vi "Set Speed.vi"(8 "error in (no error)":errorcluster, 10 "speed":dbl, 11 "VICI Settings":T1) -> (0 "error out":errorcluster, 1 "Connection Error":bool, 3 "VICI Settings":T1)   [LabVIEW 2018, in "VICI M50 Party Mode.lvlib"]
uses:
  VICI M50 Party Mode.lvlib
  Settings Cluster.ctl
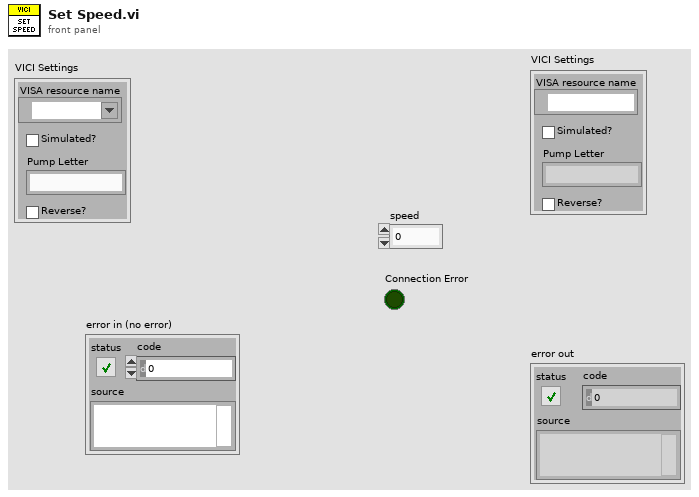
[diagram p1: front panel]
types:
  T1 = typedef "VICI M50 Party Mode.lvlib/Settings Cluster.ctl" = cluster{"VISA resource name":refnum<visa-resource-name>, "Simulated?":bool, "Pump Letter":string, "Reverse?":bool}
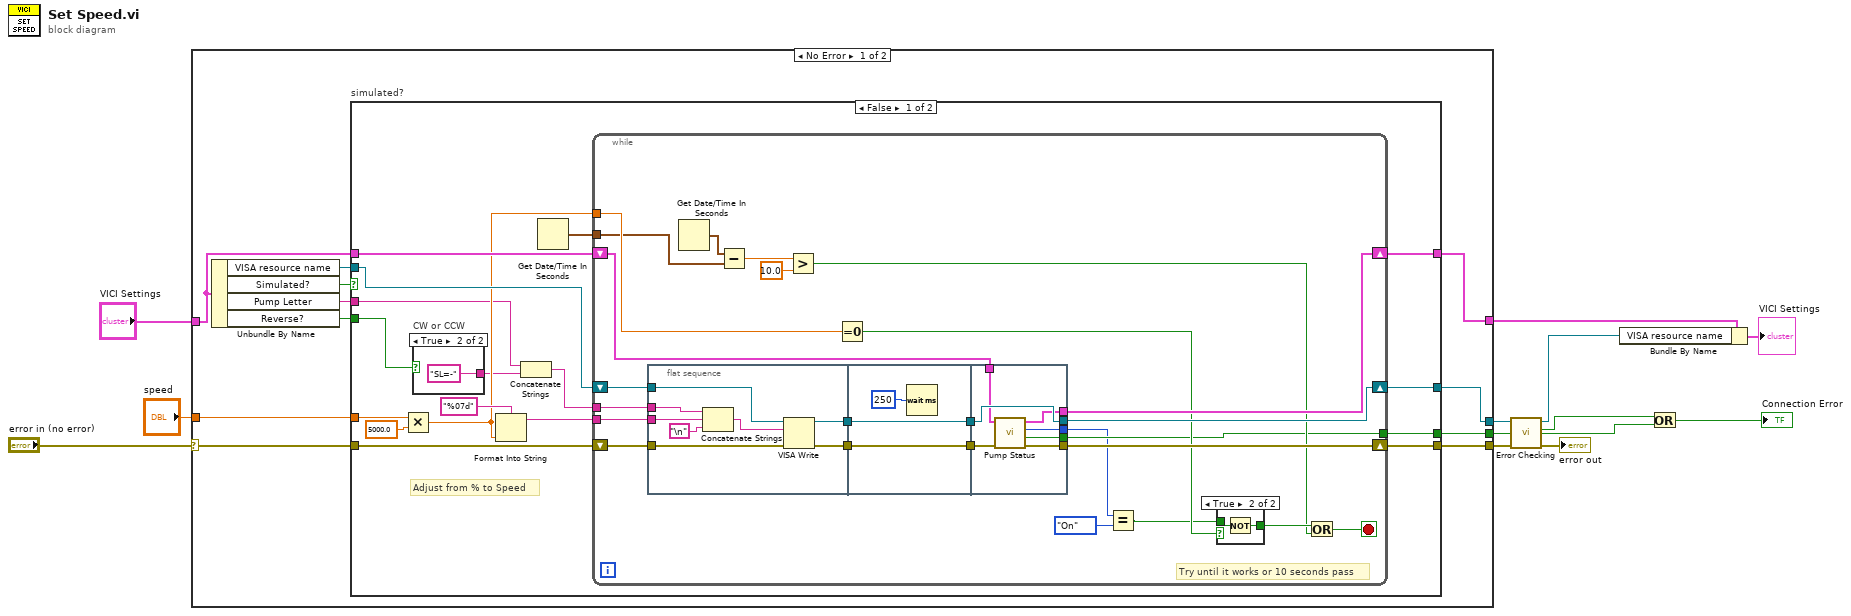
[diagram p0: block diagram]
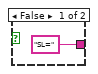
[diagram p3: hidden frame]
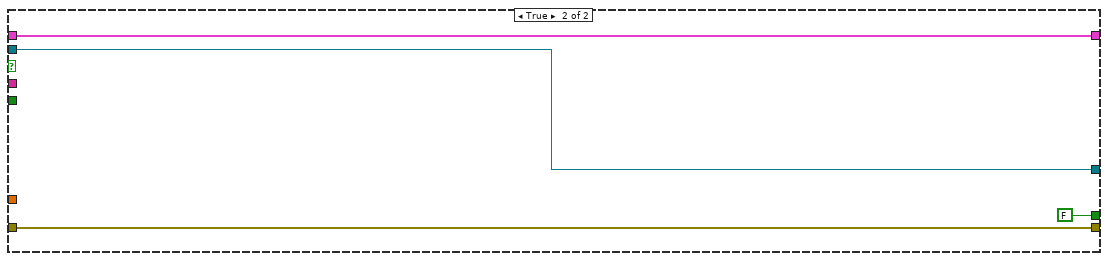
[diagram p4: hidden frame]
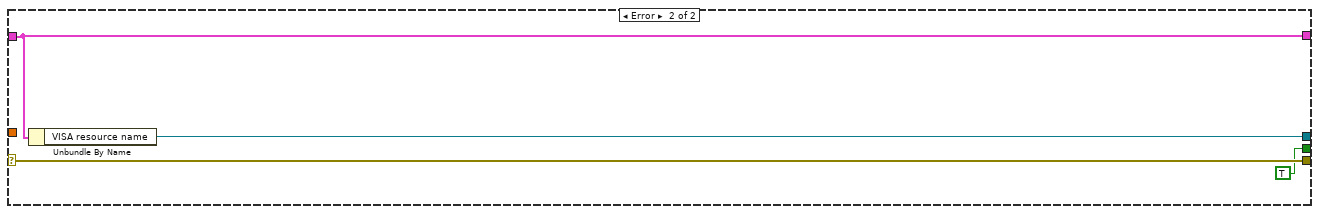
[diagram p5: hidden frame]
diagram:
  n1 = case shown="No Error" "error in (no error)" {
    selector: "error in (no error)" -> [w20 w96]
    tunnel: [w15 w95] -> w5
    tunnel: "VICI Settings" -> [w16 w95]
    tunnel: "speed" -> [w19 _]
    tunnel: [w18 w94] -> w9
    tunnel: [w17 w96] -> w8
    tunnel: [w14 TRUE ("Connection Error")] -> w3
    frame No Error {
      n2 = Unbundle By Name(w16) -> ("VISA resource name"=w22:refnum<visa-resource-name>, "Simulated?"=w21:bool, "Pump Letter"=w13:string, "Reverse?"=w23:bool)
      n3 = case "simulated?" shown="False" w21 {
        tunnel: [w38 w92] -> w18
        tunnel: w22 -> [w40 w92]
        tunnel: w20 -> [w39 w91]
        tunnel: [w37 w91] -> w17
        tunnel: w23 -> [w36 _]
        tunnel: w19 -> [w34 _]
        tunnel: w16 -> [w31 w90]
        tunnel: [w30 w90] -> w15
        tunnel: [w27 FALSE ("Connection Error")] -> w14
        tunnel: w13 -> [w24 _]
        frame False {
          # "Adjust from % to Speed"
          n4 = Multiply(x=w34, y=5000.0) -> (x*y=w29:dbl)
          n5 = case "CW or CCW" shown="True" w36 {
            tunnel: ["SL=" ("string") "SL=-" ("string")] -> w26
            frame False {
            }
            frame True {
            }
          }
          n6 = Format Into String(format string="%07d", w29) -> (resulting string=w33:string)  [unwired: 2 in, 1 out]
          n7 = Concatenate Strings(w24, w26) -> (w25:string)
          n8 = Get Date/Time In Seconds() -> (seconds since 1Jan1904=w28:timestamp)
          n9 = while {
            tunnel: w25 -> [w58]
            tunnel: w33 -> [w57]
            shift-right: [w60] -> w38
            shift-left: w40 -> [w45]
            shift-right: [w59] -> w37
            shift-left: w39 -> [w61]
            shift-right: [w55] -> w30
            shift-left: w31 -> [w56]
            tunnel: w29 -> [w54]
            tunnel: w28 -> [w47]
            tunnel: [w44] -> w27
            stop <- w50 stop-if-true
            # "Try until it works or 10 seconds pass"
            n10 = flat-sequence {
              tunnel: w45 -> [w76]
              tunnel: w61 -> [w75]
              tunnel: w58 -> [w72]
              tunnel: w57 -> [w71]
              tunnel: [w74] -> w65
              tunnel: [w73] -> w64
              tunnel: w65 -> [w79]
              tunnel: w64 -> [w78]
              tunnel: [w79] -> w63
              tunnel: [w78] -> w62
              tunnel: [w84] -> w59
              tunnel: [w86] -> w60
              tunnel: w63 -> [w86]
              tunnel: w62 -> [w85]
              tunnel: w56 -> [w83]
              tunnel: [w82] -> w55
              tunnel: [w81] -> w43
              tunnel: [w80] -> w44
              frame #0 {
                n11 = Concatenate Strings(w72, w71, "\n") -> (w70:string)
                n12 = VISA Write(VISA resource name=w76, write buffer=w70, error in (no error)=w75) -> (VISA resource name out=w74:refnum<visa-resource-name>, error out=w73:errorcluster)  [unwired: 1 out]
              }
              frame #1 {
                n13 = Wait (ms)(milliseconds to wait=u32 250) -> ()  [unwired: 1 out]
              }
              frame #2 {
                n14 = call "Pump Status.vi"("error in (no error)"=w85, "VICI Settings"=w83) -> ("error out"=w84:errorcluster, "Connection Error"=w80:bool, "Pump On?"=w81:enum16{"Off", "On", "Not Initialized"}, "VICI Settings"=w82:T1)  [unwired: 6 in]
              }
            }
            n15 = Get Date/Time In Seconds() -> (seconds since 1Jan1904=w46:timestamp)
            n16 = Subtract(x=w46, y=w47) -> (x-y=w52:dbl)
            n17 = Greater?(x=w52, y=10.0) -> (0:w48:bool)
            n18 = Equal To 0?(x=w54) -> (x = 0?=w53:bool)
            n19 = Equal?(x=w43, y=enum16{"Off", "On", "Not Initialized"}."On") -> (x = y?=w42:bool)
            n20 = case shown="True" w53 {
              tunnel: [w66 w68] -> w51
              tunnel: w42 -> [w66 w67]
              frame False {
              }
              frame True {
                n21 = Not(x=w67) -> (.not. x?=w68:bool)
              }
            }
            n22 = Or(x=w51, y=w48) -> (x .or. y?=w50:bool)
          }
        }
        frame True {
        }
      }
    }
    frame Error {
      n23 = Unbundle By Name(w95) -> ("VISA resource name"=w94:refnum<visa-resource-name>)
    }
  }
  n24 = call "Error Checking.vi"("error in (no error)"=w8, "VISA resource name"=w9) -> ("error out"=→"error out":errorcluster, "Connection Error"=w2:bool, "VISA resource name"=w6:refnum<visa-resource-name>)  [unwired: 7 in]
  n25 = Bundle By Name(cluster=w5, "VISA resource name"=w6) -> (→"VICI Settings":T1)
  n26 = Or(x=w2, y=w3) -> (x .or. y?=→"Connection Error":bool)
